vi "Get Final Time Value.vi"   [LabVIEW 2018]
doc: "返回<B>波形输入</B>中的结束时间值。 使用的公式为：xf = x0 + <B>波形输入</B>的持续时间。 通过连线数据至<B>波形输入</B>输入端可确定要使用的多态实例，也可手动选择实例。"
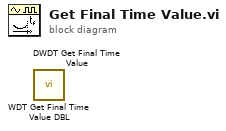
[diagram p0: block diagram]
diagram:
  n1 = call "WDT Get Final Time Value DBL.vi"() -> ()  [unwired: 9 in, 3 out]
  n2 = call "DWDT Get Final Time Value.vi"() -> ()  [unwired: 9 in, 3 out]
